vi "setOutputGain.vi"(8 "error in (no error)":errorcluster, 10 "OutputGain":dbl[](array[numeric]), 11 "Instrument.LockinAPI in":refnum<class "Instrument.LockinAPI.lvclass">) -> (0 "error out":errorcluster, 3 "Instrument.LockinAPI out":refnum<class "Instrument.LockinAPI.lvclass">)   [LabVIEW 2019, in "Instrument.LockinAPI.lvclass"]
doc: "API to put lockin into remote mode.\n\nIf address=\"\", this API reads from localhost\nIf address is remote lockin, you need to add this computer to allowed whitelist on the lockin computer you are trying to access."
uses:
  Instrument.LockinAPI.lvclass
  C:/Users/patrick/Documents/GitHub/Instrument-Framework/lvsrc/Instrument/Instrument.lvclass
  Typedefs/API/LockinAPI.Commands--Enum.ctl
  16b0612a-153c-498e-8e8b-4591927cf31d.vi
  16b0612a-153c-498e-8e8b-4591927cf31d.vi/3101038e-18df-4964-a0bc-afb85091a795.vi
  16b0612a-153c-498e-8e8b-4591927cf31d.vi/3101038e-18df-4964-a0bc-afb85091a795.vi/4418f206-fb4e-407e-af6a-5fb285b6dcf4.vi
  16b0612a-153c-498e-8e8b-4591927cf31d.vi/3101038e-18df-4964-a0bc-afb85091a795.vi/bcf99e2d-fa5e-49f0-8a0c-cc251a993aa0.vi
  16b0612a-153c-498e-8e8b-4591927cf31d.vi/3101038e-18df-4964-a0bc-afb85091a795.vi/172b7090-e3f6-491c-a96b-76c52b69cbb3.vi
  <vilib>/JDP Science/JSONtext/Make JSON Array.vi
  16b0612a-153c-498e-8e8b-4591927cf31d.vi/3101038e-18df-4964-a0bc-afb85091a795.vi/bcf99e2d-fa5e-49f0-8a0c-cc251a993aa0.vi/dedd4cad-c96b-4b0f-81d7-757a4f62e9c2.vi
  16b0612a-153c-498e-8e8b-4591927cf31d.vi/3101038e-18df-4964-a0bc-afb85091a795.vi/172b7090-e3f6-491c-a96b-76c52b69cbb3.vi/b49d99f2-4547-44f6-b072-2d03dddf974f.vi
  16b0612a-153c-498e-8e8b-4591927cf31d.vi/3101038e-18df-4964-a0bc-afb85091a795.vi/172b7090-e3f6-491c-a96b-76c52b69cbb3.vi/308b7a6a-8d18-4990-b4e9-3a4e25bf6449.vi
  Instrument/API/Enum to String.vi
  Instrument/Private/Get RC Connection Status.vi
  <vilib>/JDP Science/JSONtext/Variant to JSON Text.vi
  <vilib>/JDP Science/JSONtext/support/Format JSON Array Text.vi
  Instrument/API/Send and Receive.vi
  <vilib>/JDP Science/JSONtext/JSON text to Variant.vi
  <vilib>/Utility/Data Type/Get Type Information.vi
  <vilib>/JDP Science/JSONtext/LVClass Serializer/JSONtext LVClass Serializer.lvclass
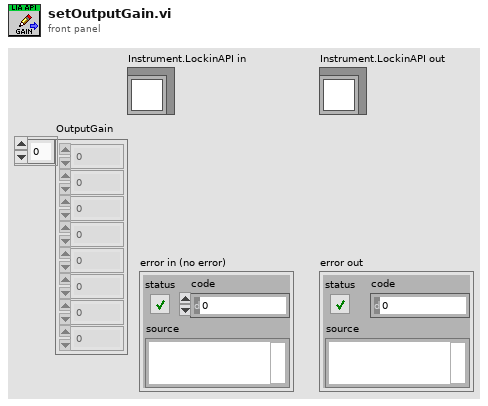
[diagram p1: front panel]
types:
  T1 = typedef "Instrument.LockinAPI.lvclass/LockinAPI.Commands--Enum.ctl" = enum16{"setAI", "setAO", "setAO_Amplitude", "setAO_DC", "setAO_Frequency", "setAO_Phase", "setAO_Function", "setAO_I+", "setREF", "setREF_Frequency", "setREF_Phase", "setREF_TC", "setREF_Roll-Off", "setDAQ", "setSampling", "setOffset", "setState", "getState", "getAO", "getAI", "getResults", "getSampling", "getAOconfig", "getREFconfig", "setInputGain", "setOutputGain", "getInputGain", "getOutputGain", "setSamplingMode", "getSamplingMode", "setSweep", "setSweepTime", "setSweepTable", "getStatus", "getSweepResults", "getSweepWaveforms", "startSweep", "stopSweep", "setAUX", "getAUX"}
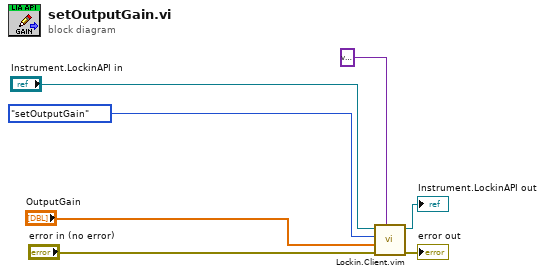
[diagram p0: block diagram]
diagram:
  n1 = call "Lockin.Client.vim"("Data Out type"=variant, "error in (no error)"="error in (no error)", "Data"="OutputGain", "Command"=LockinAPI.Commands--Enum."setOutputGain", "Instrument.LockinAPI in"="Instrument.LockinAPI in") -> ("error out"=→"error out":errorcluster, "Instrument.LockinAPI out"=→"Instrument.LockinAPI out":refnum<class "Instrument.LockinAPI.lvclass">)  [unwired: 4 in, 1 out]
